vi "initialise.vi"(8 "error in (no error)":errorcluster, 11 "ImagingModeDL090130Frame in":refnum<class "ImagingModeDL090130Frame.lvclass">=refnum) -> (0 "error out":errorcluster, 3 "ImagingModeDL090130Frame out":refnum<class "ImagingModeDL090130Frame.lvclass">)   [LabVIEW 2010, in "ImagingModeDL090130Frame.lvclass"]
doc: "The dynamic dispatch-version of this VI initalises the plug-in object by allocating and initalising any dynamic resources need."
uses:
  ImagingModeDL090130Frame.lvclass
  ImagingModeDL090923Scaffold/ImagingModeDL090923Scaffold/ImagingModeDL090923Scaffold.lvclass
  common/xcontrols/XIntensityCompensation/XIntensityCompensation/XIntensityCompensation.xctl
  Instrument/GenericInstrument/GenericInstrument/GenericInstrument.lvclass
  DAQ/GenericDAQ/GenericDAQ/GenericDAQ.lvclass
  Display/GenericDisplay/GenericDisplay/GenericDisplay.lvclass
  Analyser/GenericAnalyser/GenericAnalyser/GenericAnalyser.lvclass
  ScanHead/GenericScanHead/GenericScanHead/GenericScanHead.lvclass
  Stimulator/GenericStimulator/GenericStimulator/GenericStimulator.lvclass
  common/classes/ErrorController/ErrorController/class_data.vi
  common/classes/ErrorController/ErrorController/ErrorController.lvclass
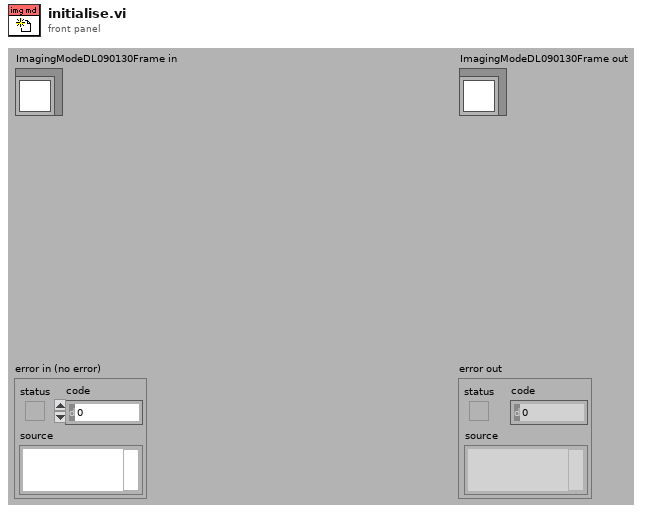
[diagram p1: front panel]
types:
  T1 = enum8{"Enabled", "Disabled", "Disabled and Grayed Out"}
  T2 = typedef "controls_refs.ctl" = cluster{"scan start button":refnum<vi>, "tabs":cluster{"main":refnum<vi>, "settings":refnum<vi>}, "subpanels":cluster{"imagingMode":refnum<vi>, "scanHead":refnum<vi>, "display":refnum<vi>, "experimentController":refnum<vi>, "instrument":refnum<vi>, "stage":refnum<vi>, "stimulator":refnum<vi>, "dataCollection":refnum<vi>, "analyser":refnum<vi>, "daq":refnum<vi>, "imageAssembler":refnum<vi>}, "drop-downs":cluster{"run mode":refnum<vi>, "imagingMode":refnum<vi>, "experimentalController":refnum<vi>, "objective":refnum<vi>}, "status lights":cluster{"experimentController":refnum<vi>, "imagingMode":refnum<vi>, "scanHead":refnum<vi>, "daq":refnum<vi>, "imageAssembler":refnum<vi>, "dataCollection":refnum<vi>, "display":refnum<vi>, "analyser":refnum<vi>, "stage":refnum<vi>, "stimulator":refnum<vi>, "instrument":refnum<vi>}, "message":refnum<vi>, "stimulator enabled?":refnum<vi>, "saving":cluster{"data folder path":refnum<vi>, "file base name":refnum<vi>, "notebook":refnum<vi>}, "progress bar":refnum<vi>, "update icon":refnum<vi>, "title":refnum<vi>, "main vi":refnum<vi>, "user":refnum<vi>, "exit_button":refnum<vi>, "CPU usage %":refnum<vi>}
  T3 = typedef "ImagingModeDL090130Frame.lvclass/control_refs.ctl" = cluster{"resolution controls":cluster{"x pixels":refnum<vi>, "y pixels":refnum<vi>, "ratio x factor":refnum<vi>, "ratio y factor":refnum<vi>}, "speed controls":cluster{"pixel dwell time":refnum<vi>, "line scan time":refnum<vi>, "frame rate":refnum<vi>}, "number of frames controls":cluster{"# of frames":refnum<vi>, "duration":refnum<vi>, "# of repetitions":refnum<vi>}, "current value indicators":cluster{"frame #":refnum<vi>, "repetition #":refnum<vi>, "offset":refnum<vi>}, "step controls":cluster{"step size":refnum<vi>, "return to origin?":refnum<vi>, "translation mode":refnum<vi>, "XIntensityCompensation":refnum<vi>}, "settings":refnum<vi>, "defineButton":refnum<vi>}
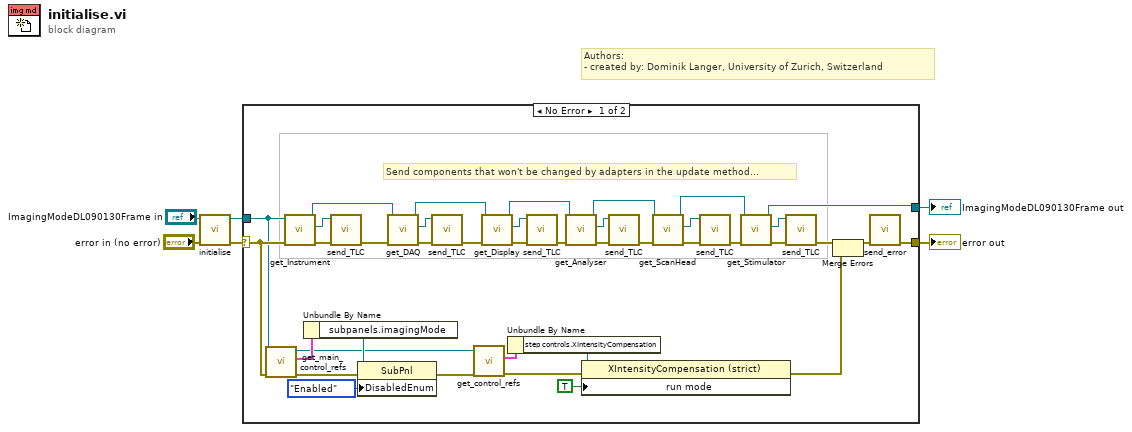
[diagram p0: block diagram]
diagram:
  # "Authors: \n- created by: Dominik Langer, University of Zurich, Switzerland"
  n1 = call-parent "initialise.vi"("error in (no error)"="error in (no error)", "GenericPlugin in"="ImagingModeDL090130Frame in") -> ("error out"=w4:errorcluster, "GenericPlugin out"=w3:refnum<class "ImagingModeDL090130Frame.lvclass">)  [unwired: 8 out]
  n2 = case shown="No Error" w4 {
    selector: w4 -> [w16 w46]
    tunnel: w3 -> [w15 w47]
    tunnel: [w20 w46] -> w2
    tunnel: [w7 w47] -> w1
    frame No Error {
      # "Send components that won't be changed by adapters in the update method..."
      n3 = call-dynamic "get_main_control_refs.vi"("error in (no error)"=w16, "GenericPlugin.lvclass in"=w15) -> ("error out"=w43:errorcluster, "control references"=w41:T2, "GenericPlugin.lvclass out"=w8:refnum<class "ImagingModeDL090130Frame.lvclass">)  [unwired: 7 out]
      n4 = call-dynamic "get_Instrument.vi"("error in (no error)"=w16, "ScanModeDL090923Scaffold in"=w15) -> ("error out"=w28:errorcluster, "Instrument"=w27:refnum<class "GenericInstrument.lvclass">, "ScanModeDL090923Scaffold out"=w24:refnum<class "ImagingModeDL090130Frame.lvclass">)  [unwired: 4 in, 3 out]
      n5 = Unbundle By Name(w41) -> ("subpanels.imagingMode"=w42:refnum<vi>)
      n6 = call-dynamic "send_TLC.vi"("error in (no error)"=w28, "GenericToplevelComponent in"=w27) -> ("error out"=w25:errorcluster)  [unwired: 8 in, 1 out]
      n7 = property class="SubPnl"(reference=w42, error in=w43, "DisabledEnum"=T1."Enabled" ("Disabled")) -> (error out=w14:errorcluster)  [unwired: 1 out]
      n8 = call-dynamic "get_DAQ.vi"("error in (no error)"=w25, "ScanModeDL090923Scaffold in"=w24) -> ("error out"=w22:errorcluster, "DAQ"=w26:refnum<class "GenericDAQ.lvclass">, "ScanModeDL090923Scaffold out"=w21:refnum<class "ImagingModeDL090130Frame.lvclass">)  [unwired: 4 in, 3 out]
      n9 = call-dynamic "send_TLC.vi"("error in (no error)"=w22, "GenericToplevelComponent in"=w26) -> ("error out"=w23:errorcluster)  [unwired: 8 in, 1 out]
      n10 = call-dynamic "get_control_refs.vi"("error in (no error)"=w14, "ImagingModeDL090130Frame in"=w8) -> ("error out"=w12:errorcluster, "control refs"=w13:T3)  [unwired: 7 in, 1 out]
      n11 = call-dynamic "get_Display.vi"("error in (no error)"=w23, "ScanModeDL090923Scaffold in"=w21) -> ("error out"=w44:errorcluster, "Display"=w45:refnum<class "GenericDisplay.lvclass">, "ScanModeDL090923Scaffold out"=w39:refnum<class "ImagingModeDL090130Frame.lvclass">)  [unwired: 7 out]
      n12 = Unbundle By Name(w13) -> ("step controls.XIntensityCompensation"=w17:refnum<vi>)
      n13 = call-dynamic "send_TLC.vi"("error in (no error)"=w44, "GenericToplevelComponent in"=w45) -> ("error out"=w40:errorcluster)  [unwired: 8 in, 1 out]
      n14 = call-dynamic "get_Analyser.vi"("error in (no error)"=w40, "ScanModeDL090923Scaffold in"=w39) -> ("error out"=w38:errorcluster, "Analyser"=w37:refnum<class "GenericAnalyser.lvclass">, "ScanModeDL090923Scaffold out"=w35:refnum<class "ImagingModeDL090130Frame.lvclass">)  [unwired: 4 in, 3 out]
      n15 = property class="XIntensityCompensation (strict)"(reference=w17, error in=w12, "run mode"=TRUE ("free-run mode")) -> (error out=w10:errorcluster)  [unwired: 1 out]
      n16 = call-dynamic "send_TLC.vi"("error in (no error)"=w38, "GenericToplevelComponent in"=w37) -> ("error out"=w36:errorcluster)  [unwired: 8 in, 1 out]
      n17 = call-dynamic "get_ScanHead.vi"("error in (no error)"=w36, "ScanModeDL090923Scaffold in"=w35) -> ("error out"=w32:errorcluster, "ScanHead"=w30:refnum<class "GenericScanHead.lvclass">, "ScanModeDL090923Scaffold out"=w29:refnum<class "ImagingModeDL090130Frame.lvclass">)  [unwired: 4 in, 3 out]
      n18 = call-dynamic "send_TLC.vi"("error in (no error)"=w32, "GenericToplevelComponent in"=w30) -> ("error out"=w31:errorcluster)  [unwired: 8 in, 1 out]
      n19 = call-dynamic "get_Stimulator.vi"("error in (no error)"=w31, "ScanModeDL090923Scaffold in"=w29) -> ("error out"=w34:errorcluster, "Stimulator"=w33:refnum<class "GenericStimulator.lvclass">, "ScanModeDL090923Scaffold out"=w7:refnum<class "ImagingModeDL090130Frame.lvclass">)  [unwired: 4 in, 3 out]
      n20 = call-dynamic "send_TLC.vi"("error in (no error)"=w34, "GenericToplevelComponent in"=w33) -> ("error out"=w11:errorcluster)  [unwired: 8 in, 1 out]
      n21 = Merge Errors(w11, w10) -> (w9:errorcluster)
      n22 = call "send_error.vi"("error in (no error)"=w9) -> ("error out"=w20:errorcluster)  [unwired: 10 in]
    }
    frame Error {
    }
  }
  "error out" <- w2
  "ImagingModeDL090130Frame out" <- w1
